vi "Dark Array FGV.vi"(10 "Control":enum16{"get", "add", "reset"}(ring), 11 "New Dark In":dbl[][](array[numeric])) -> (3 "Out":dbl[][](array[numeric]))   [LabVIEW 2013, in "AvaSpec.lvlib"]
uses:
  avantesSpectrometer/AvaSpec.lvlib
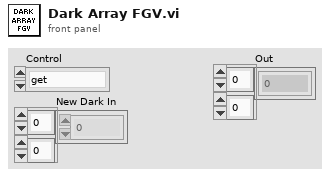
[diagram p1: front panel]
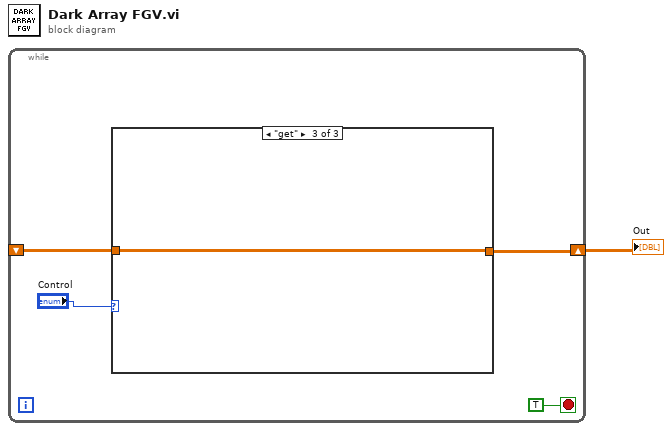
[diagram p0: block diagram]
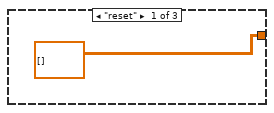
[diagram p2: hidden frame]
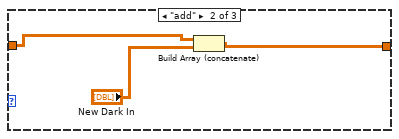
[diagram p3: hidden frame]
diagram:
  n1 = while {
    shift-right: [w3] -> w1
    shift-left: _ -> [w2]
    stop <- TRUE stop-if-true
    n2 = case shown="\"get\"" "Control" {
      tunnel: [dbl[][] [] w7 w10] -> w3
      tunnel: w2 -> [_ w9 w10]
      frame "reset" {
      }
      frame "add" {
        n3 = Build Array (concatenate)(w9, "New Dark In") -> (w7:dbl[][])
      }
      frame "get" {
      }
    }
  }
  "Out" <- w1
